vi "客户机.vi"() -> ()   [LabVIEW 2017]
panel:
  out "数字":i32
  in  "停止":bool
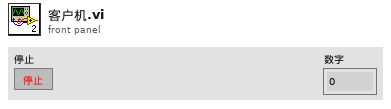
[diagram p1: front panel]
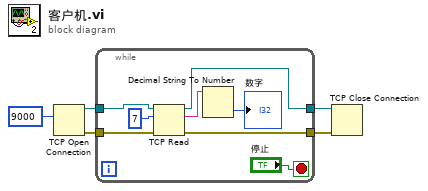
[diagram p0: block diagram]
diagram:
  n1 = TCP Open Connection(remote port or service name=u16 9000 ("远程端口或服务名称")) -> (connection ID=w5:refnum<k5>, error out=w4:errorcluster)  [unwired: 4 in]
  n2 = while {
    tunnel: w5 -> [w12]
    tunnel: w4 -> [w11]
    tunnel: [w10] -> w3
    tunnel: [w9] -> w2
    stop <- "停止" stop-if-true
    n3 = TCP Read(connection ID=w12, bytes to read=7 ("读取的字节"), error in (no error)=w11) -> (connection ID out=w10:refnum<k5>, data out=w7:string, error out=w9:errorcluster)  [unwired: 2 in]
    n4 = Decimal String To Number(string=w7) -> (number=→"数字":i32)  [unwired: 2 in, 1 out]
  }
  n5 = TCP Close Connection(connection ID=w3, error in (no error)=w2) -> ()  [unwired: 1 in, 2 out]
